vi "SLL DE AI Moving Average V1.0.vi"(8 "error in (no error)":errorcluster, 9 "Window Size":i32=3 min=1 max=1000 step=1, 11 "Array":dbl[][](array[numeric])) -> (0 "error out":errorcluster, 3 "Average Array":dbl[][](array[numeric]))   [LabVIEW 2009]
doc: "Calculates the moving average of te data for the specified window size.\n\nRPF. Yogesh.\n\nCopyright © 2007, Soliton Technologies.\nAll rights reserved."
panel:
  # "Moving Average"
  # "Inputs"
  # "Output"
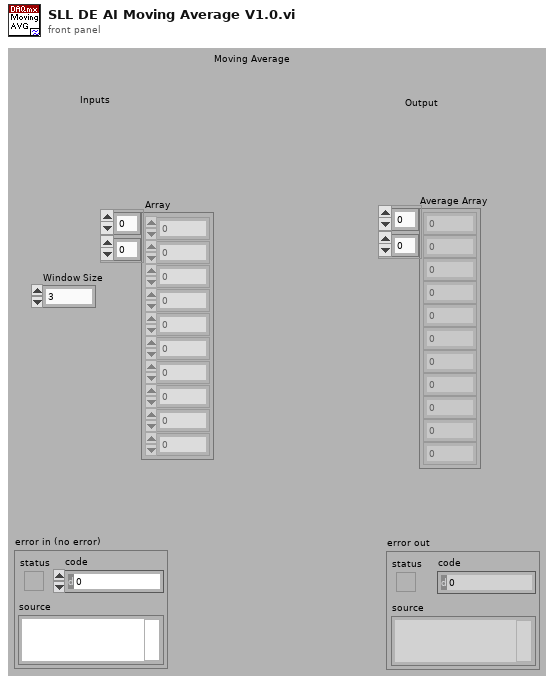
[diagram p1: front panel]
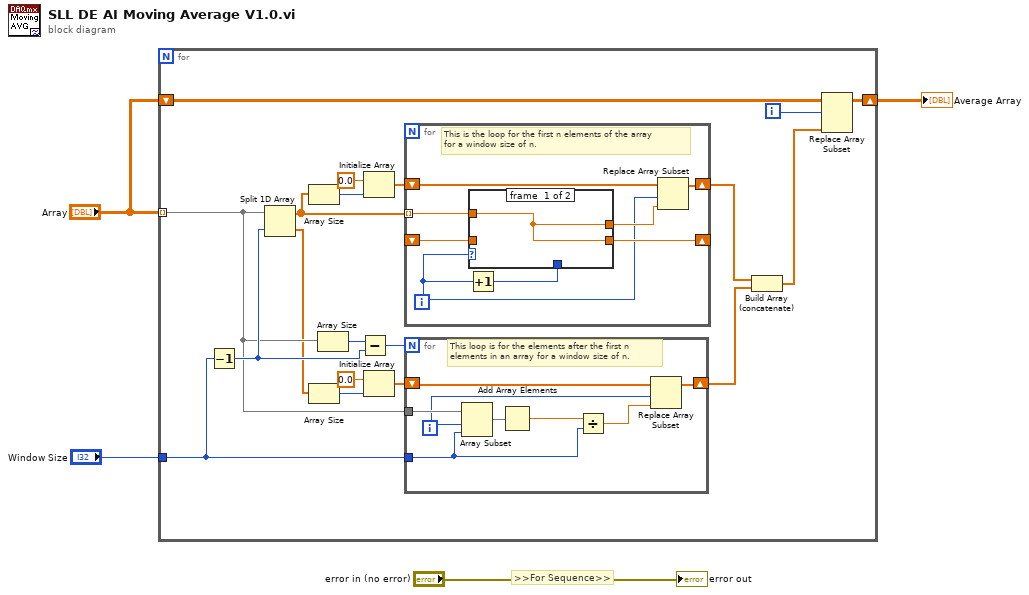
[diagram p0: block diagram]
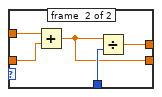
[diagram p2: hidden frame]
diagram:
  # ">>For Sequence>>"
  n1 = for {
    tunnel: "Array" -> [w22] mode=indexing
    tunnel: "Window Size" -> [w21]
    shift-right: [w7] -> w2
    shift-left: "Array" -> [w6]
    i -> [w5]
    n2 = Decrement(x=w21) -> (x-1=w23:i32)
    n3 = Split 1D Array(array=w22, index=w23) -> (first subarray=w13:dbl[], second subarray=w9:dbl[])
    n4 = Array Size(array=w13) -> (size(s)=w14:i32)
    n5 = Array Size(array=w9) -> (size(s)=w12:i32)
    n6 = Array Size(array=w22) -> (size(s)=w20:i32)
    n7 = Subtract(x=w20, y=w23) -> (x-y=w19:i32)
    n8 = Initialize Array(0.0 ("element"), w14) -> (w16:dbl[])
    n9 = Initialize Array(0.0 ("element"), w12) -> (w10:dbl[])
    n10 = for {
      shift-right: [w38] -> _
      shift-left: _ -> [w32]
      shift-right: [w37] -> w18
      shift-left: w16 -> [w36]
      tunnel: w13 -> [w33] mode=indexing
      i -> [w34]
      # "This is the loop for the first n elements of the array\nfor a window size of n."
      n11 = Increment(x=w34) -> (x+1=w39:i32)
      n12 = case shown="-1, Default" w34 {
        tunnel: w39 -> [_ w45]
        tunnel: [w40 w44] -> w38
        tunnel: [w40 w43] -> w35
        tunnel: w33 -> [w40 w42]
        tunnel: w32 -> [_ w41]
        frame #0 {
        }
        frame #1 {
          n13 = Add(x=w42, y=w41) -> (x+y=w44:dbl)
          n14 = Divide(x=w44, y=w45) -> (x/y=w43:dbl)
        }
      }
      n15 = Replace Array Subset(array=w36, new element=w35, index=w34) -> (w37:dbl[])
    }
    n16 = for {
      N: w19 -> [_]
      tunnel: w22 -> [w31]
      tunnel: w21 -> [w28]
      shift-right: [w25] -> w17
      shift-left: w10 -> [w24]
      i -> [w27]
      # "This loop is for the elements after the first n\nelements in an array for a window size of n."
      n17 = Array Subset(array=w31, index=w27, length=w28) -> (w30:dbl[])
      n18 = Add Array Elements(numeric array=w30) -> (sum=w29:dbl)
      n19 = Divide(x=w29, y=w28) -> (x/y=w26:dbl)
      n20 = Replace Array Subset(array=w24, new element=w26, index=w27) -> (w25:dbl[])
    }
    n21 = Build Array (concatenate)(w18, w17) -> (w8:dbl[])
    n22 = Replace Array Subset(array=w6, new element=w8, index (row)=w5) -> (w7:dbl[][])  [unwired: 1 in]
  }
  "Average Array" <- w2
  "error out" <- "error in (no error)"
